vi "JSONconfig_DCPowerSupplyArray.vi"(2 "error in (no error)":errorcluster, 3 "String":string, 4 "DCPowerInformationClusterArray_Input":T1[](array[typedef])) -> (0 "error out":errorcluster, 1 "DCPowerInformationClusterArray out":T1[](array[typedef]))   [LabVIEW 2019]
uses:
  Controls/DCPowerBlock_byInstrument_Control.ctl
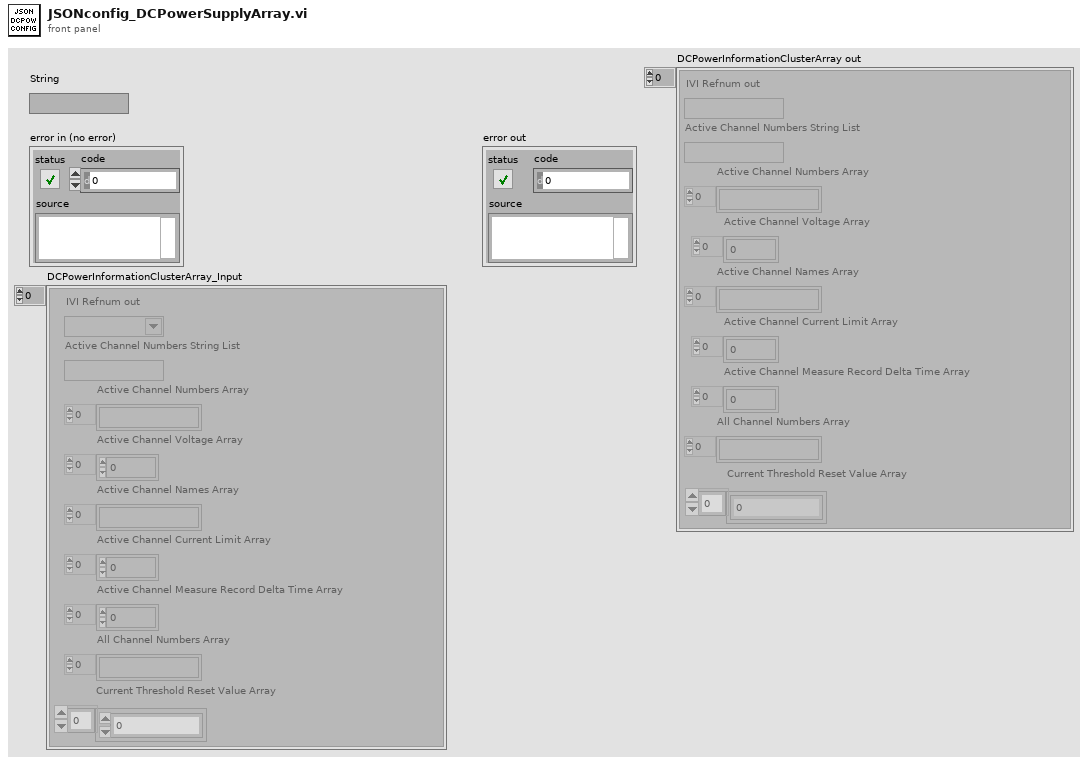
[diagram p1: front panel]
types:
  T1 = typedef "DCPowerBlock_byInstrument_Control.ctl" = cluster{"IVI Refnum out":refnum<k15>, "Active Channel Numbers String List":string, "Active Channel Numbers Array":string[], "Active Channel Voltage Array":dbl[], "Active Channel Names Array":string[], "Active Channel Current Limit Array":dbl[], "Active Channel Measure Record Delta Time Array":dbl[], "All Channel Numbers Array":string[], "Current Threshold Reset Value Array":dbl[]}
  T2 = cluster{"IVI Refnum out":refnum<k15>, "Active Channel Numbers String List":string, "Active Channel Numbers Array":string[], "Active Channel Voltage Array":dbl[], "Active Channel Names Array":string[], "Active Channel Current Limit Array":dbl[], "Active Channel Measure Record Delta Time Array":dbl[], "All Channel Numbers Array":string[]}[]
  T3 = cluster{"Supply_Number":dbl, "Supply_Array":cluster{"instr_name":string, "voltage":dbl, "supply_name":string, "channel":string, "current_clamp":dbl, "measure_record_length":dbl, "aperature_time":dbl, "current_reset_value_A":dbl}[]}
  T4 = cluster{"instr_name":string, "voltage":dbl, "supply_name":string, "channel":string, "current_clamp":dbl, "measure_record_length":dbl, "aperature_time":dbl, "current_reset_value_A":dbl}[]
  T5 = cluster{"instrument handle out":refnum<k15>, "channel":string, string[], dbl[], string[], dbl[], dbl[], string[], dbl[]}
  T6 = cluster{"IVI Refnum out":refnum<k15>, string, "Active Channel Numbers Array":string[], "Active Channel Voltage Array":dbl[], "Active Channel Names Array":string[], "Active Channel Current Limit Array":dbl[], "Active Channel Measure Record Delta Time Array":dbl[], "All Channel Numbers Array":string[], "Current Threshold Reset Value Array":dbl[]}
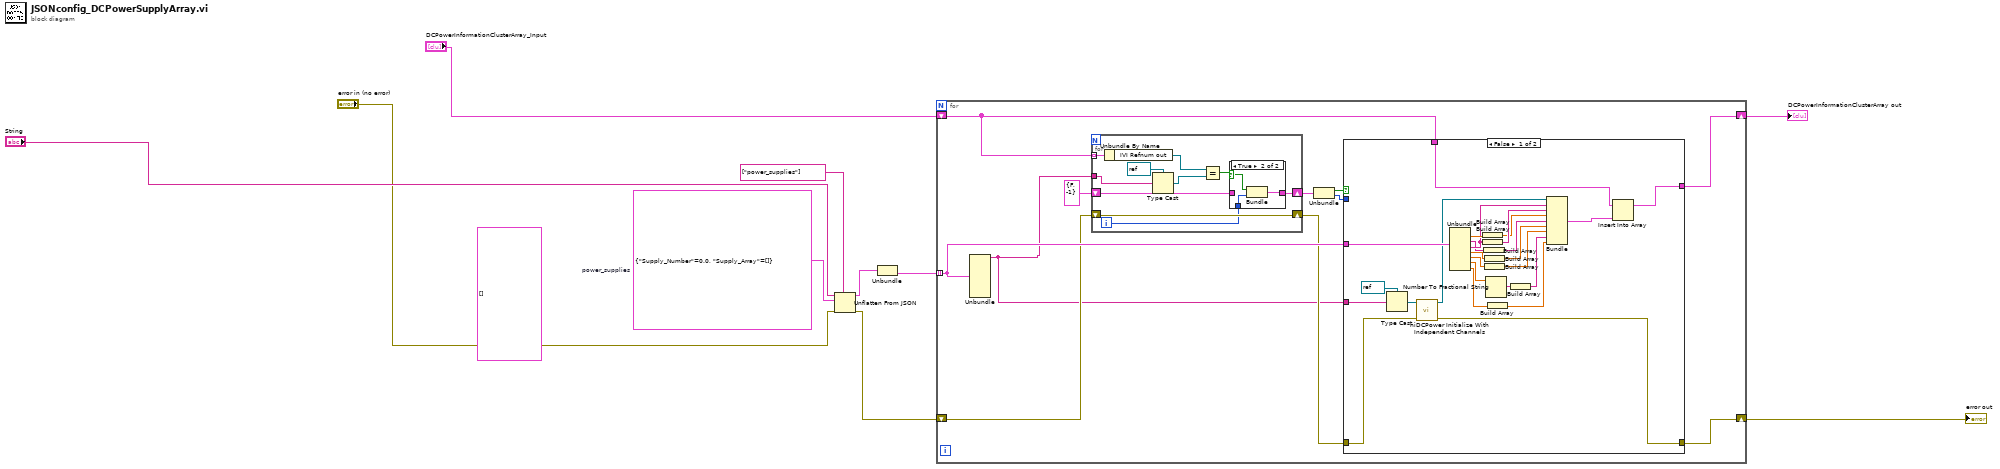
[diagram p0: block diagram]
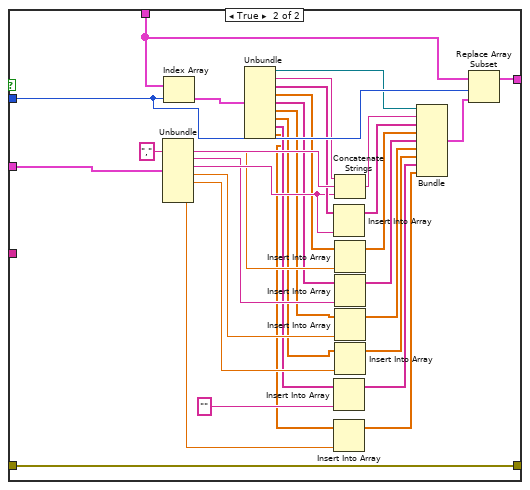
[diagram p3: hidden frame]
diagram:
  (unwired) T2 [] ("DCPowerInformationClusterArray_Input in")
  w5 = T3 {"Supply_Number"=0.0, "Supply_Array"=[]}  # power_supplies
  n1 = Unflatten From JSON(path=string[] ["power_supplies"], JSON string="String", type and defaults=w5, error in (no error)="error in (no error)") -> (value=w7:T3, error out=w9:errorcluster)  [unwired: 3 in]
  n2 = Unbundle(w7) -> ("Supply_Array"=w8:T4)  [unwired: 1 out]
  n3 = for {
    tunnel: w8 -> [w20] mode=indexing
    shift-right: [w19] -> w1
    shift-left: "DCPowerInformationClusterArray_Input" -> [w18]
    shift-right: [w14] -> w10
    shift-left: w9 -> [w12]
    n4 = Unbundle(w20) -> ("instr_name"=w11:string)  [unwired: 7 out]
    n5 = for {
      tunnel: w11 -> [w23]
      shift-right: [w30] -> w13
      shift-left: w12 -> [w30]
      tunnel: w18 -> [w29] mode=indexing
      shift-right: [w26] -> w16
      shift-left: cluster{bool, i32} {FALSE, -1} -> [w27]
      i -> [w25]
      n6 = Unbundle By Name(w29) -> ("IVI Refnum out"=w28:refnum<k15>)
      n7 = Type Cast(type=refnum<k15> refnum ("resource name"), x=w23) -> (*(type *) &x=w22:refnum<k15>)
      n8 = Equal?(x=w28, y=w22) -> (x = y?=w31:bool)
      n9 = case shown="True" w31 {
        selector: w31 -> [_ w33]
        tunnel: w27 -> [w32 _]
        tunnel: [w32 w35] -> w26
        tunnel: w25 -> [_ w34]
        frame False {
        }
        frame True {
          n10 = Bundle(w33, w34) -> (w35:cluster{bool, i32})  [unwired: 1 in]
        }
      }
    }
    n11 = Unbundle(w16) -> (w21:bool, w15:i32)
    n12 = case shown="False" w21 {
      tunnel: w20 -> [w60 w92]
      tunnel: [w48 w72] -> w19
      tunnel: w18 -> [w47 w90]
      tunnel: w15 -> [_ w89]
      tunnel: [w42 w64] -> w14
      tunnel: w13 -> [w43 w64]
      tunnel: w11 -> [w44 _]
      frame False {
        n13 = Type Cast(type=refnum<k15> refnum ("resource name"), x=w44) -> (*(type *) &x=w45:refnum<k15>)
        n14 = call <instrlib>:"niDCPower Initialize With Independent Channels.vi"("error in (no error)"=w43, "resource name"=w45) -> ("error out"=w42:errorcluster, "instrument handle out"=w41:refnum<k15>)  [unwired: 8 in]
        n15 = Unbundle(w60) -> ("voltage"=w59:dbl, "supply_name"=w55:string, "channel"=w58:string, "current_clamp"=w53:dbl, "measure_record_length"=w51:dbl, "aperature_time"=w40:dbl, "current_reset_value_A"=w37:dbl)  [unwired: 1 out]
        n16 = Build Array(w59) -> (w56:dbl[])
        n17 = Build Array(w58) -> (w57:string[])
        n18 = Build Array(w55) -> (w54:string[])
        n19 = Build Array(w53) -> (w52:dbl[])
        n20 = Build Array(w51) -> (w50:dbl[])
        n21 = Number To Fractional String(number=w40) -> (F-format string=w39:string)  [unwired: 3 in]
        n22 = Build Array(w37) -> (w36:dbl[])
        n23 = Build Array(w39) -> (w38:string[])
        n24 = Bundle("instrument handle out"=w41, "channel"=w58, w57, w56, w54, w52, w50, w38, w36) -> (w49:T5)  [unwired: 1 in]
        n25 = Insert Into Array(array=w47, new element=w49) -> (w48:T1[])  [unwired: 1 in]
      }
      frame True {
        n26 = Unbundle(w92) -> ("voltage"=w80:dbl, "supply_name"=w78:string, "channel"=w83:string, "current_clamp"=w77:dbl, "measure_record_length"=w76:dbl, "current_reset_value_A"=w63:dbl)  [unwired: 2 out]
        n27 = Index Array(array=w90, index=w89) -> (element=w91:T1)
        n28 = Unbundle(w91) -> ("IVI Refnum out"=w88:refnum<k15>, "Active Channel Numbers String List"=w86:string, "Active Channel Numbers Array"=w84:string[], "Active Channel Voltage Array"=w81:dbl[], "Active Channel Names Array"=w79:string[], "Active Channel Current Limit Array"=w69:dbl[], "Active Channel Measure Record Delta Time Array"=w68:dbl[], "All Channel Numbers Array"=w75:string[], "Current Threshold Reset Value Array"=w62:dbl[])
        n29 = Insert Into Array(array=w84, new element=w83) -> (w82:string[])  [unwired: 1 in]
        n30 = Insert Into Array(array=w75, new element="" ("new element/subarray")) -> (w66:string[])  [unwired: 1 in]
        n31 = Insert Into Array(array=w62, new element=w63) -> (w61:dbl[])  [unwired: 1 in]
        n32 = Concatenate Strings(w86, "," ("string"), w83) -> (w85:string)
        n33 = Insert Into Array(array=w81, new element=w80) -> (w73:dbl[])  [unwired: 1 in]
        n34 = Insert Into Array(array=w79, new element=w78) -> (w71:string[])  [unwired: 1 in]
        n35 = Insert Into Array(array=w69, new element=w77) -> (w70:dbl[])  [unwired: 1 in]
        n36 = Insert Into Array(array=w68, new element=w76) -> (w67:dbl[])  [unwired: 1 in]
        n37 = Bundle("IVI Refnum out"=w88, w85, "Active Channel Numbers Array"=w82, "Active Channel Voltage Array"=w73, "Active Channel Names Array"=w71, "Active Channel Current Limit Array"=w70, "Active Channel Measure Record Delta Time Array"=w67, "All Channel Numbers Array"=w66, "Current Threshold Reset Value Array"=w61) -> (w65:T6)  [unwired: 1 in]
        n38 = Replace Array Subset(array=w90, new element=w65, index=w89) -> (w72:T1[])
      }
    }
  }
  "error out" <- w10
  "DCPowerInformationClusterArray out" <- w1
